vi "chaim_Tx_back_to host.vi"() -> ()   [LabVIEW 2021]
doc: "Acquires data from the Rx ports and streams the data to the host while receiving data from the host and generating the resulting waveform at the Tx ports of the NI USRP-294x/295x device. Use this VI as a template for the Simple NI-USRP Streaming sample project."
uses:
  <instrlib>/_niInstr/Register Bus/v1/FPGA/Public/Read Cmd Data.ctl
  <vilib>/Platform/TimedLoop/XDataNode/timing_clust.ctl
  <vilib>/Platform/TimedLoop/XDataNode/nitl_modes.ctl
  <vilib>/Platform/TimedLoop/XDataNode/wakeup.ctl
  <instrlib>/_niInstr/DSP/v1/Shared/Public/IQ Data.ctl
  <vilib>/rvi/Emulation/niFpgaSctlEmulationGetInTimedLoop.vi
  <vilib>/rvi/Emulation/niFpgaEmulationReportErrorSimple.vi
  <vilib>/rvi/Emulation/niFpgaGetClockAttributes.vi
  <vilib>/rvi/Emulation/niFpgaCriticalErrorInLSC.vi
  <instrlib>/_niInstr/DSP/v1/FPGA/Public/Sub VIs/Data Conversion/IQ to I16 - 1 spc - S18.1.vi
  <vilib>/rvi/interface/RandomDataEmulation/nirviRandomDataMultiElementFPGAFIFO.vi
  <instcachedir>/0/nirviRandomDataMultiElementFPGAFIFO_3E9965BA1FAD4E7B8DABA31768A09B1F.lvgen/nirviRandomDataMultiElementFPGAFIFO_3E9965BA1FAD4E7B8DABA31768A09B1F_001.vi
  <vilib>/rvi/interface/RandomDataEmulation/niFpgaRandomDataHandleErrors.vi
  <instrlib>/_niInstr/Basic Elements/v1/FPGA/Private/Count Up U8.vi
  <vilib>/rvi/eio/common/nirviEmuTemplateMethod_errors.vi
  <vilib>/Platform/TimedLoop/XDataNode/XDataNode.xnode
  <vilib>/rvi/DataTransferAndStorage/Container/XNode/niFpgaContainer.xnode
  <vilib>/rvi/interface/RandomDataEmulation/nirviRandomDataFpgaMultiElementTemplate.vi
  <vilib>/rvi/interface/RandomDataEmulation/nirviRandomDataFpgaReadWriteTemplate.vi
  <vilib>/eio/EIONode/EIONode.xnode
  <vilib>/Platform/TimedLoop/XDataNode/XDNodeRunTimeDep.lvlib
  <instrlib>/_niInstr/Register Bus/v1/FPGA/niInstr Register Bus v1 FPGA.lvlib
  <instrlib>/niUsrpRio/Config/v1/FPGA/niUsrpRio Config v1 FPGA.lvlib
  <instrlib>/_niInstr/DSP/v1/Shared/niInstr DSP v1 Shared.lvlib
  <instrlib>/_niInstr/DSP/v1/FPGA/niInstr DSP v1 FPGA.lvlib
  <instrlib>/_niInstr/Basic Elements/v1/FPGA/niInstr Basic Elements v1 FPGA.lvlib
panel:
  in  "dcimator":u8
  in  "LED/RF 1/TX1 RX1":enum8{"Off", "Green", "Red", "Amber"}(ring)
  in  "LED/RF 0/TX1 RX1":enum8{"Off", "Green", "Red", "Amber"}(ring)
  out "tx free":bool[](array[boolean])
  out "pulse transmitted":u32
  out "fpga clock":u64
  in  "reset system clock":bool
  in  "RF 1/Tx/Enable":bool
  in  "RF 1/Rx/Enable":bool
  in  "RF 0/Tx/Enable":bool
  in  "RF 0/Rx/Enable":bool
  in  "reg.host read.go rcvd 0":bool
  out "reg.notify host.go 0":bool
  in  "reg.notify host.go rcvd 0":bool
  out "reg.host read.data 0":T1
  in  "reg.reset 0":bool
  # "USRP RIO pulse Streaming FPGA"
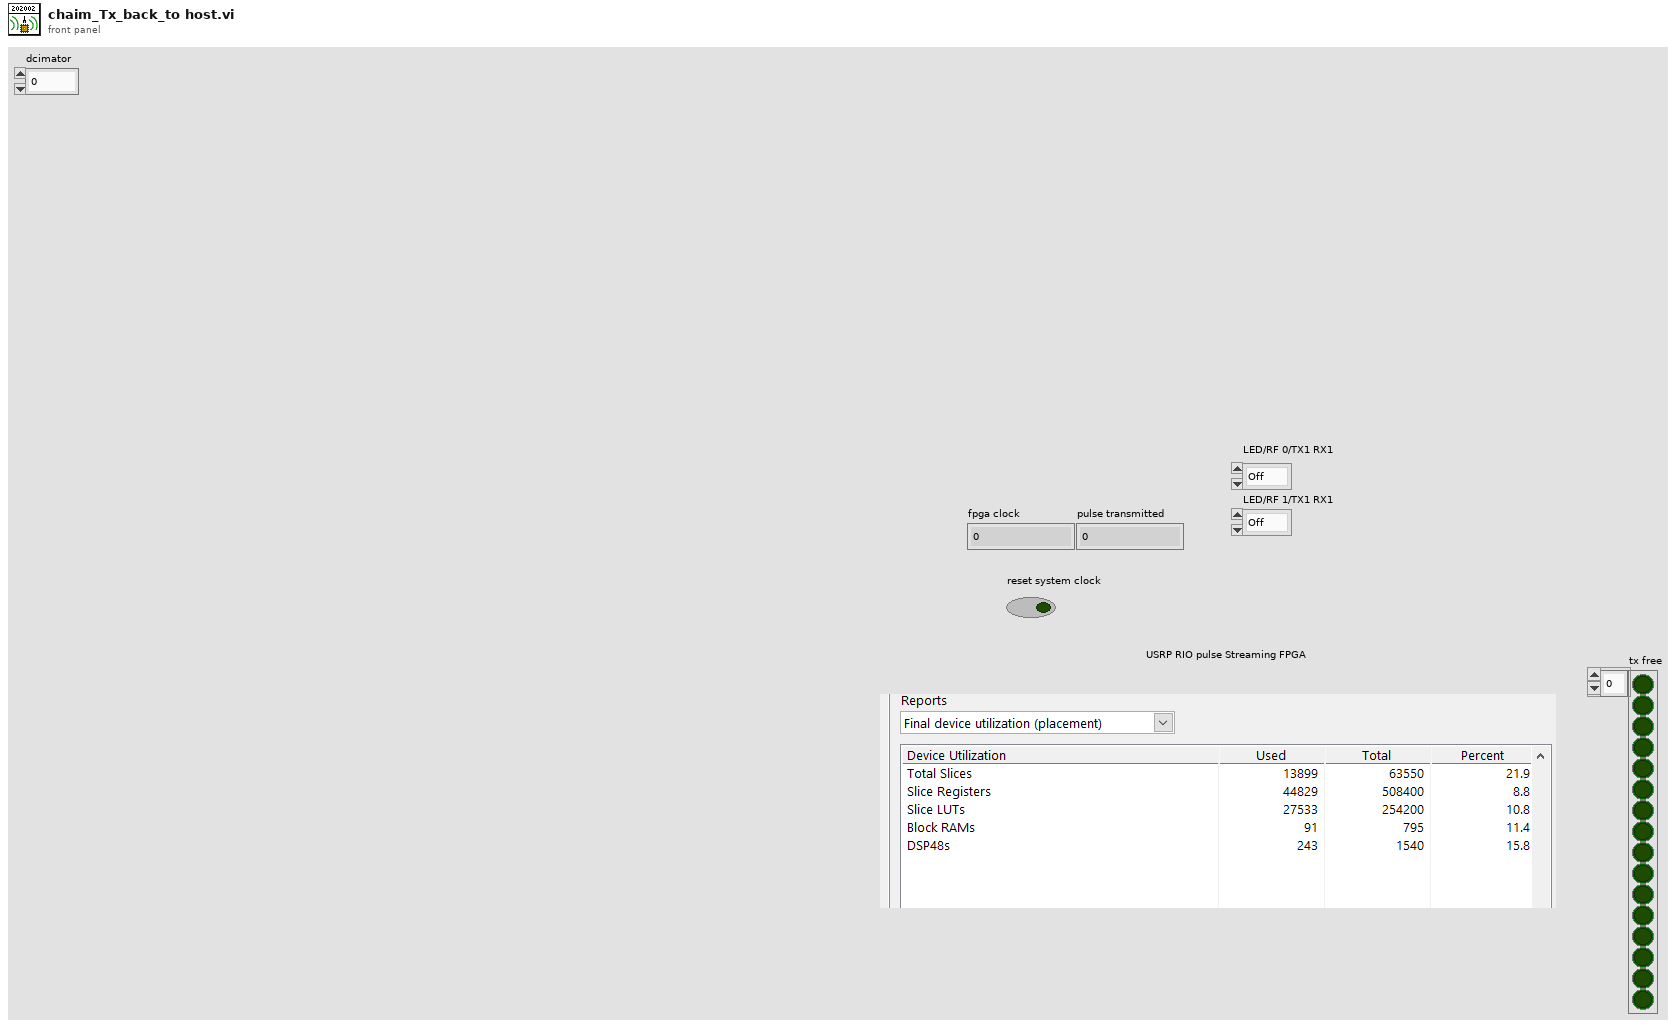
[diagram p1: front panel]
types:
  T1 = typedef "niInstr Register Bus v1 FPGA.lvlib/Read Cmd Data.ctl" = cluster{"go":bool, "data":u32}
  T2 = typedef "XDNodeRunTimeDep.lvlib/timing_clust.ctl" = cluster{"Expected End [f-1]":u64, "Actual End [f-1]":u64, "Finished Late? [f-1]":bool, "Expected End [i-1]":u64, "Actual End [i-1]":u64, "Finished Late? [i-1]":bool, "Expected Start [i]":u64, "Actual Start [i]":u64, "Expected Start [f]":u64, "Actual Start [f]":u64, "Source Name":string, "Structure Name":string, "Period":i64, "Deadline":i64, "Offset":i64, "Start":i64, "Priority":i32, "Timeout":i32, "Mode":T3, "Wakeup Reason":T4, "Error":errorcluster, "Source Type":string, "Secondary Source Type":string, "Global End Time":u64, "Global Start Time":u64, "Frame Duration":u64, "Iteration Duration":u64, "Assigned CPU":i32, "I/O Scan Engine Mode":u32}
  T3 = typedef "XDNodeRunTimeDep.lvlib/nitl_modes.ctl" = enum32{"No Change", "Process missed periods, maintain original phase", "Discard missed periods, maintain original phase", "Process missed periods, ignore original phase", "Discard missed periods, ignore original phase"}
  T4 = typedef "XDNodeRunTimeDep.lvlib/wakeup.ctl" = enum32{"Normal", "Aborted", "Asynchronous wakeup", "Timing source error", "Timed loop error", "Timeout"}
  T5 = typedef "niInstr DSP v1 Shared.lvlib/IQ Data.ctl" = cluster{"I":fxp<+/-,18,1>, "Q":fxp<+/-,18,1>, "overflow":bool}
  T6 = cluster{"DAC FIFO Reset":refnum<k21>, "RF 0 Rx Swap IQ":refnum<k21>, "RF 0 Rx Negate I":refnum<k21>, "RF 0 Rx Negate Q":refnum<k21>, "RF 0 Rx Data Valid":refnum<k21>, "RF 0 Rx Data Ever Invalid":refnum<k21>, "clear RF 0 Rx Data Ever Invalid":refnum<k21>, "RF 0 Tx Swap IQ":refnum<k21>, "RF 0 Tx Negate I":refnum<k21>, "RF 0 Tx Negate Q":refnum<k21>, "RF 1 Rx Swap IQ":refnum<k21>, "RF 1 Rx Negate I":refnum<k21>, "RF 1 Rx Negate Q":refnum<k21>, "RF 1 Rx Data Valid":refnum<k21>, "RF 1 Rx Data Ever Invalid":refnum<k21>, "clear RF 1 Rx Data Ever Invalid":refnum<k21>, "RF 1 Tx Swap IQ":refnum<k21>, "RF 1 Tx Negate I":refnum<k21>, "RF 1 Tx Negate Q":refnum<k21>}
  T7 = typedef "niUsrpRio Synchronization v1 FPGA.lvlib/Resources.ctl" = cluster{"master":refnum<k21>, "meas.enable":refnum<k21>, "meas.ready":refnum<k21>, "meas.reset":refnum<k21>, "meas.arm":refnum<k21>, "meas.valid":refnum<k21>, "meas.value":refnum<k21>, "meas.oversample factor":refnum<k21>, "cptr":refnum<k21>, "cptr.adjust":refnum<k21>, "cptr.period":refnum<k21>}
  T8 = typedef "niUsrpRio Time v1 FPGA.lvlib/Time Resources.ctl" = cluster{"reset":refnum<k21>, "time":refnum<k21>, "time.previous cptr":refnum<k21>, "new time":refnum<k21>, "new time.when":refnum<k21>, "new time.set":refnum<k21>, "which edge of ref":refnum<k21>, "pps source":refnum<k21>, "internal pps period":refnum<k21>}
  T9 = typedef "niUsrpRio Time v1 FPGA.lvlib/Future Event Resources.ctl" = cluster{"reset":refnum<k21>, "future event.time":refnum<k21>, "future event.ready":refnum<k21>, "future event.set":refnum<k21>, "future event.clear":refnum<k21>, "future event.set in past":refnum<k21>}
  T10 = cluster{"time.resources":T8, "future event.resources":T9, "future event.resources":T9, "future event.resources":T9}
  T11 = typedef "niInstr Register Bus v1 FPGA.lvlib/Register Instruction.ctl" = cluster{"subsystem":u8, "address":u16, "data":u32, "valid":bool, "read":bool}
  T12 = typedef "niInstr Register Bus v1 FPGA.lvlib/Read Completion.ctl" = cluster{"data":u32, "valid":bool}
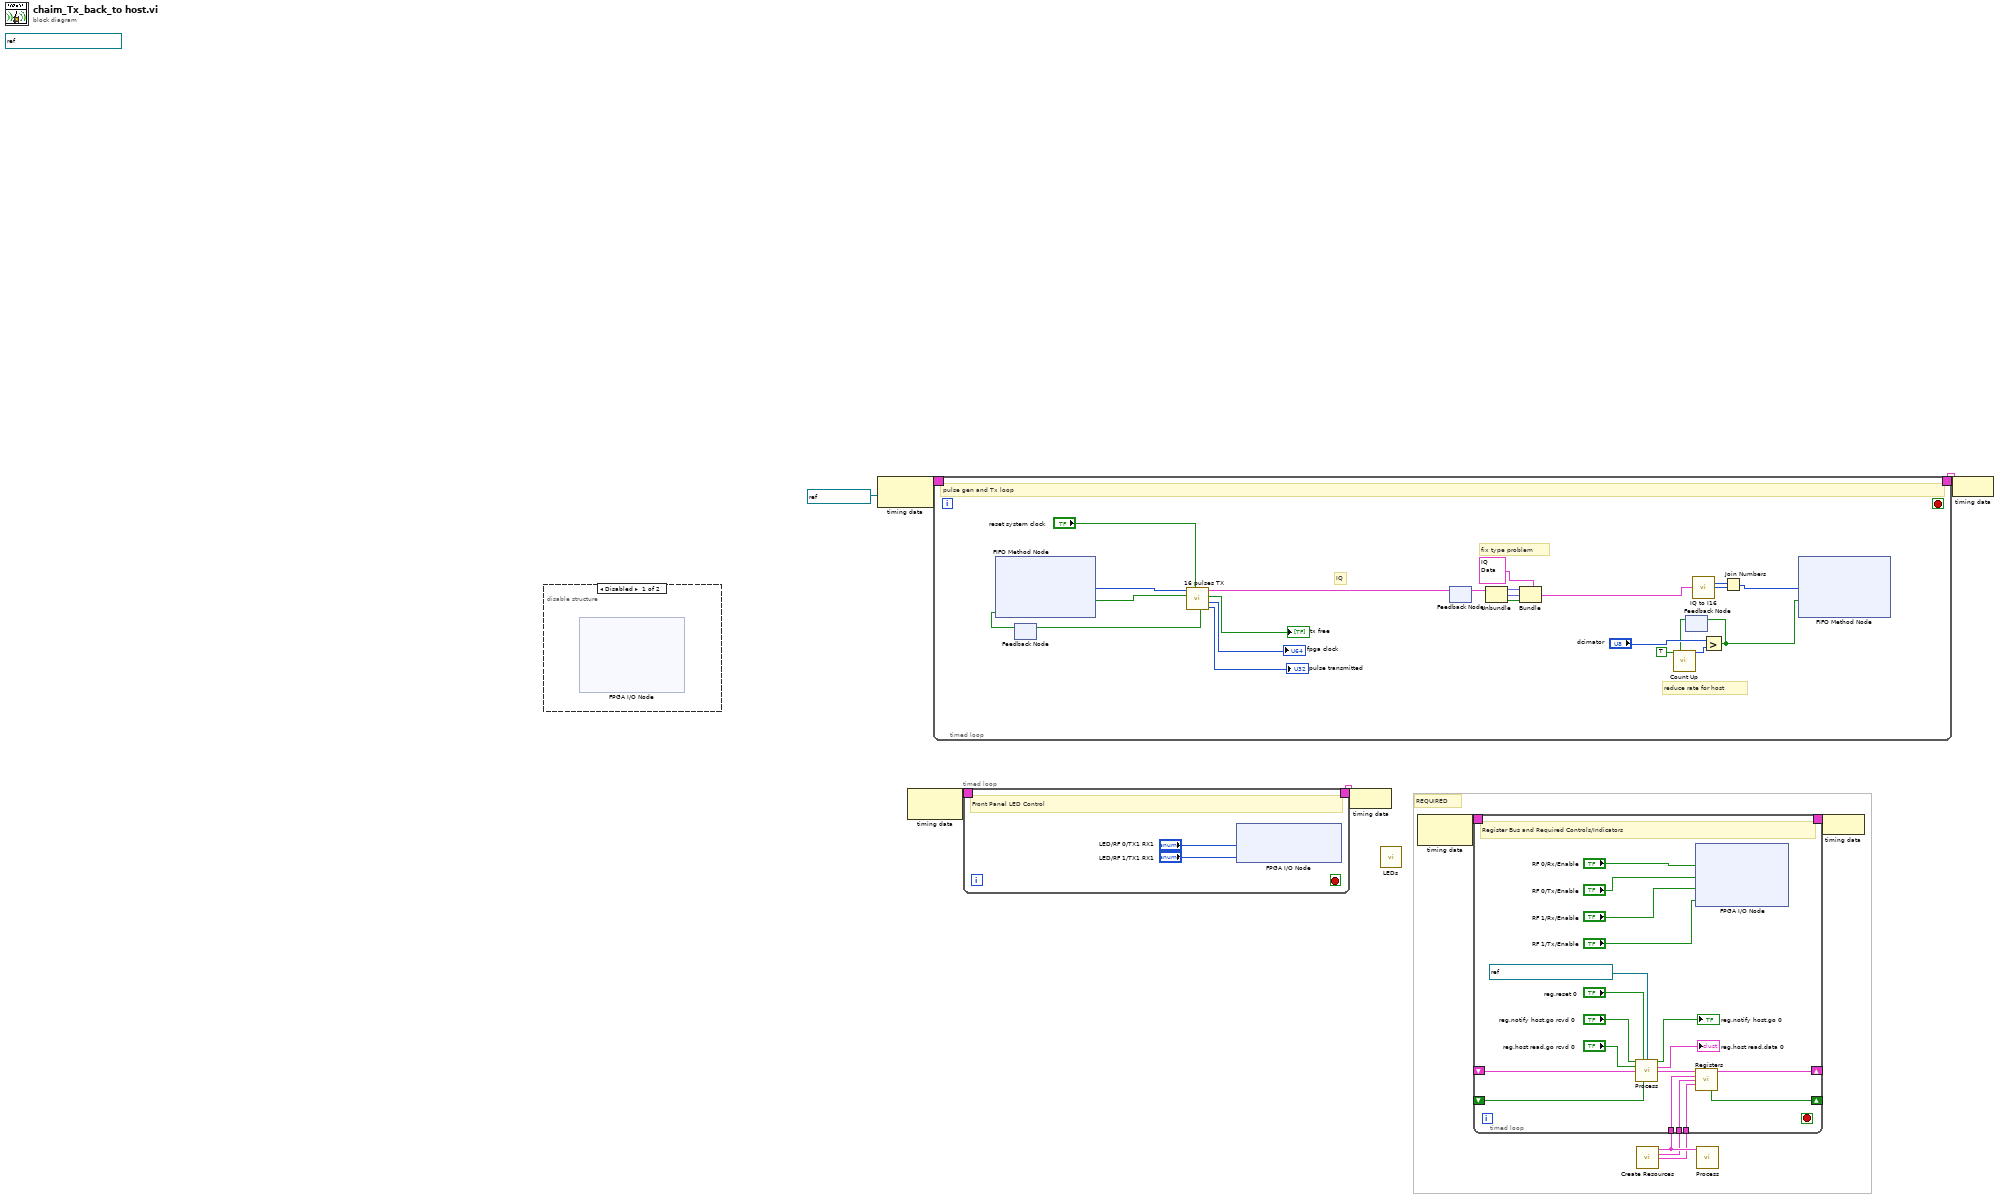
[diagram p0: block diagram]
diagram:
  (unwired) refnum<k21> "40 MHz Onboard Clock" ("Source Name")
  # "REQUIRED"
  n1 = disable-structure shown="Disabled" {
    frame Disabled {
      n2 = xnode "FPGA I/O Node"() -> ()  [unwired: 10 in, 5 out]
    }
    frame Enabled {
    }
  }
  n3 = node-c288(refnum<k21> "Data Clock" ("Source Name")) -> (w3:T2)
  n4 = node-c288() -> (w5:T2)  [unwired: 1 in]
  n5 = timed-loop {
    timing: w3 -> [_]
    timing-out: [_] -> w2
    stop <- _ stop-if-true
    # "reduce rate for host"
    # "IQ"
    # "fix type problem"
    # "pulse gen and Tx loop"
    n6 = feedback #1() -> (w29:bool)  [unwired: 1 in]
    n7 = xnode ("FIFO Method Node")("Ready for Output"=w29) -> ("Element"=w32:u64[], "Output Valid"=w33:bool)  [unwired: 1 in, 1 out]
    n8 = call "16 pulses TX.vi"("reset system clock"="reset system clock", "input Valid"=w33, "array PDW"=w32) -> ("pulse transmitted"=→"pulse transmitted":u32, "fpga clock"=→"fpga clock":u64, "tx free"=→"tx free":bool[], "RF OUT"=w20:T5, "ready for input"=w30:bool)  [unwired: 4 in]
    n9 = feedback-in #1(w30) -> ()
    n10 = feedback #2() -> (w22:T5)  [unwired: 1 in]
    n11 = feedback-in #2(w20) -> ()
    n12 = Unbundle(w22) -> ("I"=w23:fxp<+/-,18,1>, "Q"=w24:fxp<+/-,18,1>, "overflow"=w25:bool)
    n13 = Bundle(cluster=T5 {"I"=0.0, "Q"=0.0, "overflow"=FALSE} ("data in"), "I"=w23, "Q"=w24, "overflow"=w25) -> (w16:T5)
    n14 = feedback #3() -> (w12:bool)  [unwired: 1 in]
    n15 = call-poly <instrlib>:"Count Up.vi"("increment"=TRUE, "reset"=w12) -> ("count out"=w15:u8)  [unwired: 13 in]
    n16 = call-poly <instrlib>:"IQ to I16.vi"("IQ"=w16) -> ("I"=w19:i16, "Q"=w18:i16)  [unwired: 12 in, 1 out]
    n17 = Greater?(x="dcimator", y=w15) -> (0:w13:bool)
    n18 = feedback-in #3(w13) -> ()
    n19 = Join Numbers(hi=w19, lo=w18) -> ((hi.lo)=w17:u32)
    n20 = xnode ("FIFO Method Node")("Element"=w17, "Input Valid"=w13) -> ()  [unwired: 1 in, 2 out]
  }
  n21 = timed-loop {
    timing: w5 -> [_]
    timing-out: [_] -> w4
    stop <- _ stop-if-true
    # "Front Panel LED Control"
    n22 = xnode "FPGA I/O Node"("LED/RF 0/TX1 RX1"="LED/RF 0/TX1 RX1", "LED/RF 1/TX1 RX1"="LED/RF 1/TX1 RX1") -> ()  [unwired: 2 in, 2 out]
  }
  n23 = node-c288(w4) -> ()
  n24 = call "LEDs.vi"() -> ()  [unwired: 1 in]
  n25 = node-c288() -> (w10:T2)  [unwired: 1 in]
  n26 = call "Create Resources.vi"() -> ("config.resources"=w8:T6, "sync.resources"=w7:T7, "time.resources"=w6:T10)  [unwired: 13 in]
  n27 = timed-loop "Register Bus and Required Controls/Indicators" {
    timing: w10 -> [_]
    timing-out: [_] -> w9
    shift-right: [w54] -> _
    shift-left: _ -> [w53]
    shift-right: [w48] -> _
    shift-left: _ -> [w52]
    tunnel: w8 -> [w46]
    tunnel: w7 -> [w45]
    tunnel: w6 -> [w44]
    stop <- _ stop-if-true
    # "Register Bus and Required Controls/Indicators"
    n28 = call <instrlib>:"Process.vi"("reg.notify host.go rcvd"="reg.notify host.go rcvd 0", "reg.reset"="reg.reset 0", "reg.host instruction fifo"=refnum<k21> "reg.host instruction fifo 0", "reg.host read.go rcvd"="reg.host read.go rcvd 0", "read completion"=w53, "ready for output"=w52) -> ("reg.notify host.go"=→"reg.notify host.go 0":bool, "reg.host read.data"=→"reg.host read.data 0":T1, "register instruction"=w47:T11)  [unwired: 7 in]
    n29 = xnode ("FPGA I/O Node")("RF 0/Rx/Enable"="RF 0/Rx/Enable", "RF 0/Tx/Enable"="RF 0/Tx/Enable", "RF 1/Rx/Enable"="RF 1/Rx/Enable", "RF 1/Tx/Enable"="RF 1/Tx/Enable") -> ()  [unwired: 4 in, 4 out]
    n30 = call "Registers.vi"("register instruction"=w47, "config.resources"=w46, "sync.resources"=w45, "time.resources"=w44) -> ("read completion out"=w54:T12, "ready for input"=w48:bool)  [unwired: 10 in]
  }
  n31 = call <instrlib>:"Process.vi"("resources"=w8) -> ()  [unwired: 15 in]
  n32 = node-c288(w9) -> ()
  n33 = node-c288(w2) -> ()
